vi "CRYGet Value from Curve Name.vi"(10 "ML axis":u8, 11 "Level Name":string) -> (3 "Linear Value":dbl)   [LabVIEW 2013]
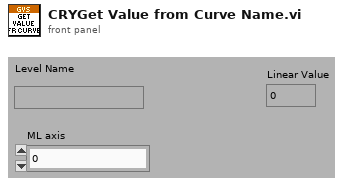
[diagram p1: front panel]
types:
  T1 = typedef "CRYData Cluster.ctl" = cluster{"Name":string, "Curve":cluster{"x":dbl, "y":dbl, "z":dbl}[], "X data":u16, "Y data":u16, "Z data":u16, "X axis":u16, "Y axis":u16, "Z axis":u16, "X unit":string, "Y unit":string, "Z unit":string, "X dB ref":dbl, "Y dB ref":dbl, "Z dB ref":dbl, "single val":bool, "protected":bool, "display X":bool, "display Y":bool, "display Z":bool, "Test Info":string, "Step No.":i32, "Plot Settings":cluster{"Color":u32, "Interpolation":u8, "Point Style":u8, "Line Style":u8, "Point Color":u32, "Line Width":u8, "Bar Plot Style":u8, "Fill To":i16}, "AutoProtect":bool}
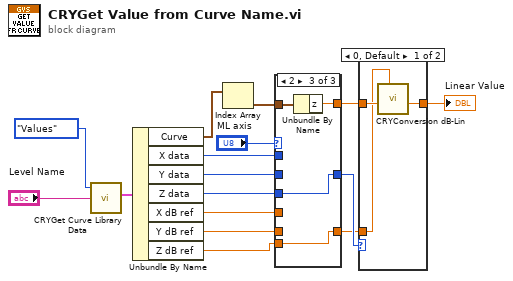
[diagram p0: block diagram]
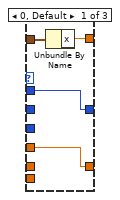
[diagram p3: hidden frame]
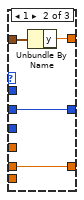
[diagram p4: hidden frame]
diagram:
  n1 = call "CRYGet Curve Library Data.vi"("Type"=enum16{"Curves", "Values", "Results", "WFM"}."Values", "Data Name"="Level Name") -> ("Value"=w15:T1)  [unwired: 4 out]
  n2 = Unbundle By Name(w15) -> ("Curve"=w14:cluster{"x":dbl, "y":dbl, "z":dbl}[], "X data"=w11:u16, "Y data"=w10:u16, "Z data"=w9:u16, "X dB ref"=w4:dbl, "Y dB ref"=w3:dbl, "Z dB ref"=w2:dbl)
  n3 = Index Array(array=w14) -> (element=w13:cluster{"x":dbl, "y":dbl, "z":dbl})  [unwired: 1 in]
  n4 = case shown="2" "ML axis" {
    tunnel: w13 -> [w20 w24 w28]
    tunnel: [w19 w23 w27] -> w12
    tunnel: w11 -> [w18 _ _]
    tunnel: w10 -> [_ w22 _]
    tunnel: w9 -> [_ _ w26]
    tunnel: [w18 w22 w26] -> w8
    tunnel: w4 -> [w17 _ _]
    tunnel: w3 -> [_ w21 _]
    tunnel: w2 -> [_ _ w25]
    tunnel: [w17 w21 w25] -> w1
    frame 0, Default {
      n5 = Unbundle By Name(w20) -> ("x"=w19:dbl)
    }
    frame 1 {
      n6 = Unbundle By Name(w24) -> ("y"=w23:dbl)
    }
    frame 2 {
      n7 = Unbundle By Name(w28) -> ("z"=w27:dbl)
    }
  }
  n8 = case shown="0, Default" w8 {
    tunnel: w12 -> [w31 w32]
    tunnel: [w30 w32] -> w5
    tunnel: w1 -> [w29 _]
    frame 0, Default {
      n9 = call "CRYConversion dB-Lin.vi"("dB ref."=w29, "Log In"=w31) -> ("Lin Out"=w30:dbl)  [unwired: 4 in, 3 out]
    }
    frame 1 {
    }
  }
  "Linear Value" <- w5
